vi "Setup.vi"(11 "Event Transport in":refnum<class "Event Transport.lvclass">) -> (0 "Error out":errorcluster, 3 "Event Transport out":refnum<class "Event Transport.lvclass">)   [LabVIEW 2025, in "jettl.lvlib" / "Transport.lvlib" / "Event Transport.lvclass"]
uses:
  Event Transport.lvclass
  Msg/Msg.lvclass
  Event Transport.lvclass/Event Transport.ctl
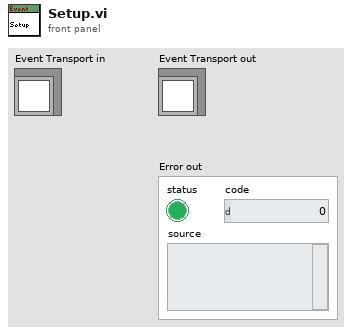
[diagram p1: front panel]
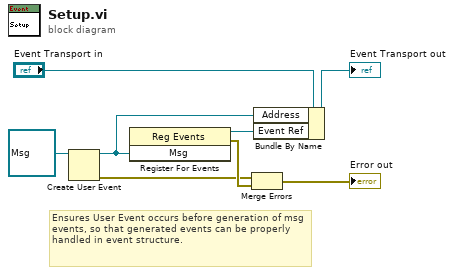
[diagram p0: block diagram]
diagram:
  # "Ensures User Event occurs before generation of msg events, so that generated events can be properly handled in event structure."
  n1 = Create User Event(user event datatype=refnum<class "Msg.lvclass"> refnum ("Msg")) -> (user event=w3:refnum<user-event>, error out=w7:errorcluster)  [unwired: 1 in]
  n2 = register-events(w3) -> (reference out=w2:refnum<event-registration>, error out=w8:errorcluster)  [unwired: 2 in]
  n3 = Merge Errors(w7, w8) -> (→"Error out":errorcluster)
  n4 = Bundle By Name(cluster="Event Transport in", "Address"=w3, "Event Ref"=w2) -> (→"Event Transport out":refnum<class "Event Transport.lvclass">)
